vi "UDP Receiver.vi"() -> ()   [LabVIEW 2009]
doc: "Use this VI with the UDP Sender VI. Run this VI first.\n\nThe UDP protocol differs from TCP in that there is no error-checking with the packets of information that are sent, and thus no guarantee whatsoever that an intended recipient will actually receive a given piece of data.\n\nUDP does offer the ability to \"broadcast\" data across a network--simply specify an IP Address of all ones (255.255.255.255) to attempt to broadcast information network-wide. Keep in mind that routers and other network hardware will generally refuse to forward the broadcast beyond certain points, so the extent of the broadcast will in practice be limited."
uses:
  UPD Xbox.ctl
  <vilib>/userDefined/High Color/nirio_resource_hc.ctl
  <vilib>/rvi/interface/nirviOpenFPGA/nirviOpenFPGA.xnode
  FPGA Bitfiles/Athena Brain.lvproj_FPGA Target 2_Combined Steering ~2D.lvbitx
  <vilib>/FPGAPlugInAG/sbRIO-9642/nirviIntfOpen_sbRIO-9642.vi
panel:
  in  "Tab Control":T1(tab)
  in  "Port":u16=61557
  out "Data Received":string
  in  "reset":bool
  out "type string":i16[](array[numeric])
  out "# of Bytes Received":i32
  in  "max bytes/read":i32=548
  out "data":T2 {"Y axis\nrotation" scale=-32700.0..32700.0; "X axis\nrotation" scale=-32700.0..32700.0; "Z axis" scale=-32700.0..32700.0; "Y axis" scale=-32700.0..32700.0; "X axis" scale=-32700.0..32700.0}
  out "error out":errorcluster
  in  "stop":bool
  # "Instructions:\n1. Open the UDP Sender.vi\n2. Make sure the Port in this VI and the Remote Port in the UDP Sender.vi are the same.\n3. Adjust the Max Bytes/Read in this VI.\n4. Run this VI first.\n5. Run the UDP Sender second.\n6. Look at the data received and the number of bytes received.\nNote: This VI is built to work with the UDP Sender.vi."
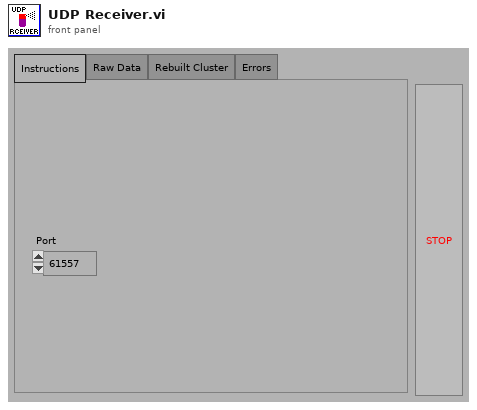
[diagram p1: front panel]
types:
  T1 = enum32{"Instructions", "Raw Data", "Rebuilt Cluster", "Errors"}
  T2 = typedef "UPD Xbox.ctl" = cluster{"B":bool, "A":bool, "Y":bool, "X":bool, "X axis":i32, "Y axis":i32, "Z axis":i32, "X axis\nrotation":i32, "Y axis\nrotation":i32, "Left Bumper":bool, "Right  Bumper":bool, "Left Thumb Button":bool, "Right Thumb Button":bool, "Stop/Back":bool, "Select":bool, "Pov Angle":i32}
  T3 = typedef "nirio_resource_hc.ctl" = tag
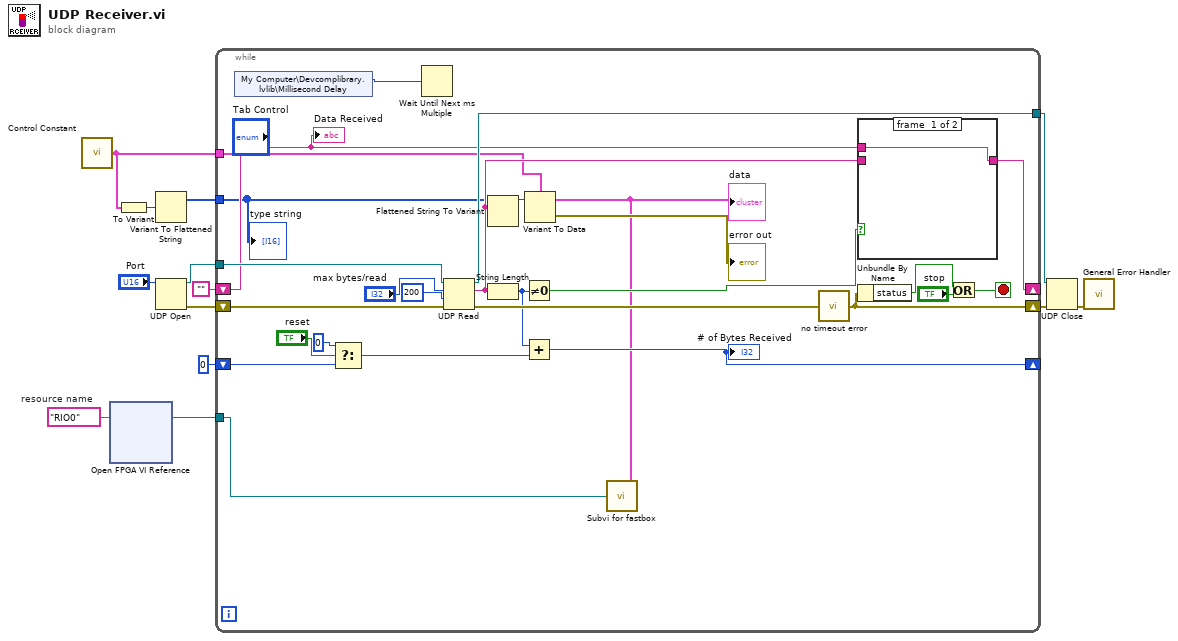
[diagram p0: block diagram]
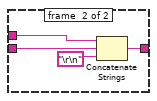
[diagram p2: hidden frame]
diagram:
  w2 = T3 "RIO0"  # resource name
  n1 = call "Control Constant.vi"() -> ("Cluster"=w3:T2)
  n2 = xnode "Open FPGA VI Reference"("resource name"=w2) -> ("FPGA VI Reference Out"=w1:refnum<k20>)  [unwired: 1 in, 1 out]
  n3 = To Variant(anything=w3) -> (Variant=w5:variant)
  n4 = Variant To Flattened String(Variant=w5) -> (1:w4:i16[])  [unwired: 1 out]
  n5 = UDP Open(11:"Port") -> (port=w11:refnum<k16>, 0:w12:errorcluster)  [unwired: 4 in, 1 out]
  n6 = while {
    shift-left: "" -> [w25]
    shift-right: [w24] -> _
    shift-left: 0 -> [w28]
    shift-right: [w30] -> _
    tunnel: [w38] -> w10
    tunnel: w11 -> [w39]
    shift-left: w12 -> [w40]
    shift-right: [w32] -> w9
    tunnel: w4 -> [w18]
    tunnel: w3 -> [w17]
    tunnel: w1 -> [w14]
    stop <- w35 stop-if-true
    n7 = shared-variable "My Computer\\Devcomplibrary.lvlib\\Millisecond Delay"() -> (w16:u32)  [unwired: 1 in, 1 out]
    n8 = Select(t=0, s="reset", f=w28) -> (s? t:f=w27:i32)
    n9 = Wait Until Next ms Multiple(millisecond multiple=w16) -> ()  [unwired: 1 out]
    n10 = UDP Read(connection ID=w39, max size (548)="max bytes/read", timeout ms (25000)=200, 8:w40) -> (data out=w21:string, error out=w33:errorcluster, 3:w38:refnum<k16>)  [unwired: 2 out]
    n11 = Flattened String To Variant(6:w21, 7:w18) -> (3:w20:variant)  [unwired: 1 in, 1 out]
    n12 = String Length(string=w21) -> (length=w23:i32)
    n13 = Not Equal To 0?(x=w23) -> (x != 0?=w22:bool)
    n14 = Add(x=w23, y=w27) -> (x+y=w30:i32)
    "# of Bytes Received" <- w30
    n15 = Variant To Data(Variant=w20, type=w17) -> (error out=→"error out":errorcluster, data=w15:T2)  [unwired: 1 in]
    "data" <- w15
    n16 = call "Subvi for fastbox.vi"("Cluster in"=w15, "FPGA VI Reference In"=w14) -> ()
    n17 = call "no timeout error.vi"("error in (no error)"=w33) -> ("error out"=w32:errorcluster)
    n18 = case shown="True" w22 {
      tunnel: w25 -> [w41 w45]
      tunnel: w21 -> [_ w43]
      tunnel: [w41 w44] -> w24
      frame #0 {
      }
      frame #1 {
        n19 = Concatenate Strings(w45, w43, "\r\n" ("Substring")) -> (w44:string)
      }
    }
    n20 = Unbundle By Name(w32) -> ("status"=w34:bool)
    n21 = Or(x=w34, y="stop") -> (x .or. y?=w35:bool)
    "Data Received" <- w25
    "type string" <- w18
  }
  n22 = UDP Close(connection ID=w10, 8:w9) -> (error out=w8:errorcluster)  [unwired: 1 out]
  n23 = call <vilib>:"General Error Handler.vi"("error in (no error)"=w8) -> ()  [unwired: 10 in, 5 out]
